vi "Test_WriteValue_InvalidRefnum_Error.vi"(8 "error in (no error)":errorcluster, 11 "TestCase in":refnum<class "TestTerminalEnabledStateBinding.lvclass">) -> (0 "error out":errorcluster, 3 "TestCase out":refnum<class "TestTerminalEnabledStateBinding.lvclass">)   [LabVIEW 2017, in "TestTerminalEnabledStateBinding.lvclass"]
uses:
  TestTerminalEnabledStateBinding.lvclass
  Source/Concrete/TerminalEnabledStateBinding/TerminalEnabledStateBinding.lvclass
  C:/Git/composed-transport/Source/ITransport/ITransport.lvclass
  Source/ITransport/ITransport.lvclass
panel:
  out "Return Error":errorcluster
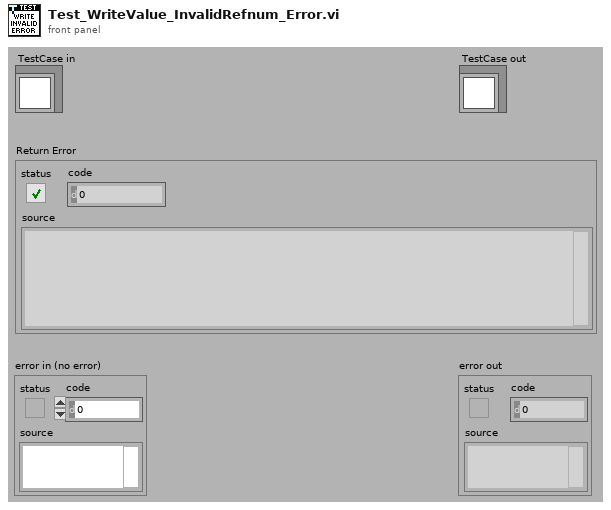
[diagram p1: front panel]
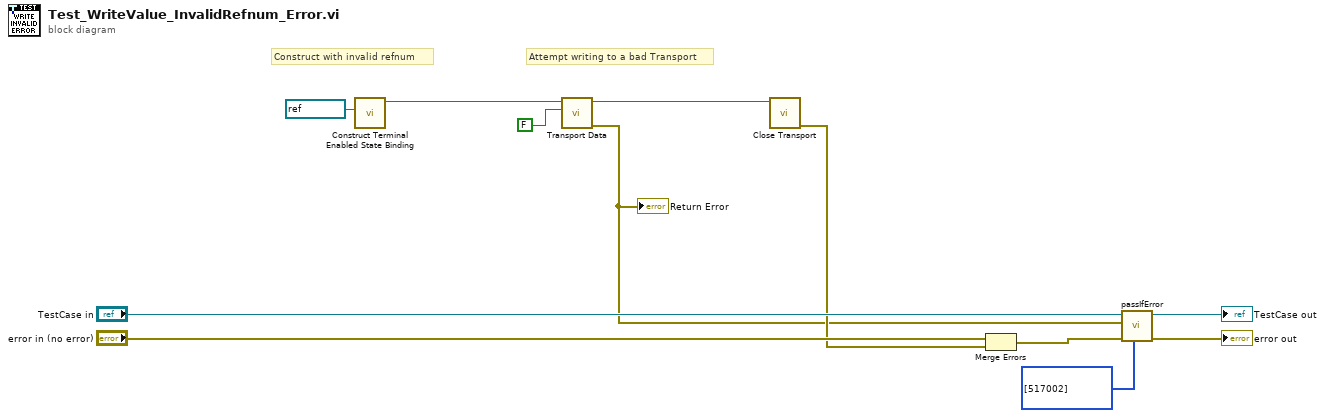
[diagram p0: block diagram]
diagram:
  # "Construct with invalid refnum"
  # "Attempt writing to a bad Transport"
  n1 = call "Construct Terminal Enabled State Binding.vi"("Control"=refnum<vi> refnum) -> ("TerminalEnabledStateBinding"=w8:refnum<class "TerminalEnabledStateBinding.lvclass">)  [unwired: 9 in, 1 out]
  n2 = call "Transport Data.vi"("Value"=FALSE, "ITransport in"=w8) -> ("error out"=w3:errorcluster, "ITransport out"=w4:refnum<class "TerminalEnabledStateBinding.lvclass">)  [unwired: 8 in]
  "Return Error" <- w3
  n3 = call-dynamic "Close Transport.vi"("ITransport in"=w4) -> ("error out"=w6:errorcluster)  [unwired: 10 in]
  n4 = Merge Errors("error in (no error)", w6) -> (w7:errorcluster)
  n5 = call-dynamic "passIfError.vi"("passing error codes (default = any error code)"=i32[] [517002], "error in (no error)"=w7, "error"=w3, "TestCase in"="TestCase in") -> ("error out"=→"error out":errorcluster, "TestCase out"=→"TestCase out":refnum<class "TestTerminalEnabledStateBinding.lvclass">)  [unwired: 6 in]
